vi "Compacting.vi"() -> ()   [LabVIEW 2019]
uses:
  JSONtext.lvlib
  c5c4e588-2033-429a-969a-39fff3336798.vi
  685e62f0-2af9-4f10-a6a8-997b7a51fd57.vi
  4d49a5eb-9da4-4064-b713-16a5944244b5.vi
panel:
  out "length":i32
  out "x = y?":bool
  out "Compacted":string
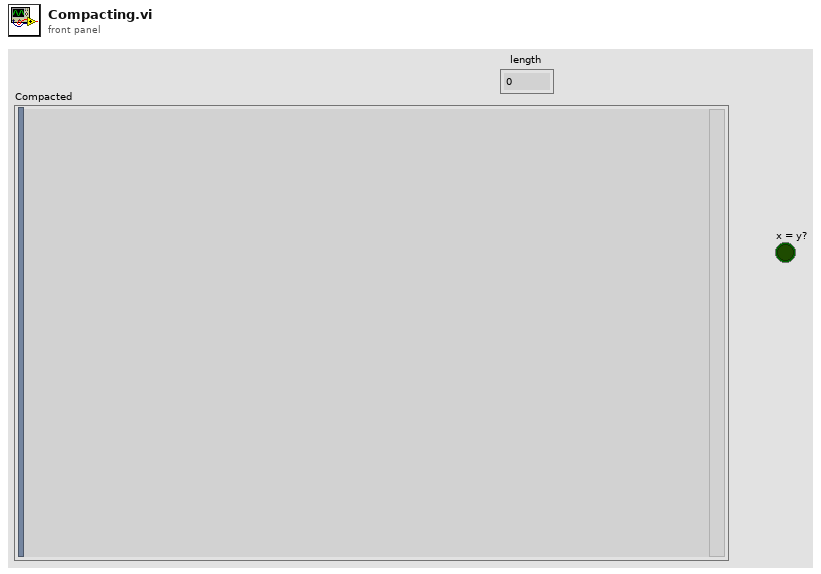
[diagram p1: front panel]
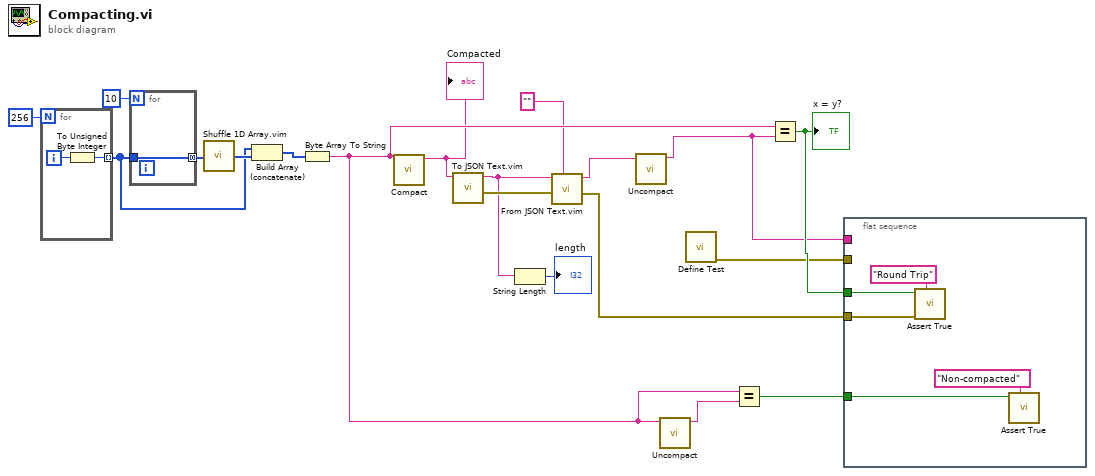
[diagram p0: block diagram]
diagram:
  n1 = for {
    N: 256 -> [_]
    tunnel: [w20] -> w4 mode=indexing
    i -> [w21]
    n2 = To Unsigned Byte Integer(number=w21) -> (unsigned 8bit integer=w20:u8)
  }
  n3 = for {
    N: 10 -> [_]
    tunnel: w4 -> [w22]
    tunnel: [w22] -> w5 mode=concatenating
  }
  n4 = call "Shuffle 1D Array.vim"("array"=w5) -> ("shuffled array"=w8:u8[])  [unwired: 4 in]
  n5 = Build Array (concatenate)(w4, w8) -> (w6:u8[])
  n6 = Byte Array To String(unsigned byte array=w6) -> (string=w16:string)
  n7 = call "Compact.vi"("Flattened Data"=w16) -> ("Compacted"=w13:string)  [unwired: 10 in]
  "Compacted" <- w13
  n8 = call "To JSON Text.vim"("Anything"=w13) -> ("error out"=w11:errorcluster, "<JSON>"=w1:string)  [unwired: 9 in]
  n9 = String Length(string=w1) -> (length=→"length":i32)
  n10 = call "From JSON Text.vim"("Data Type and Default Value"="", "error in (no error)"=w11, "JSON"=w1) -> ("error out"=w9:errorcluster, "Data out"=w12:string)  [unwired: 7 in]
  n11 = call "Uncompact.vi"("Compacted"=w12) -> ("Uncompacted"=w3:string)  [unwired: 10 in]
  n12 = call "Uncompact.vi"("Compacted"=w16) -> ("Uncompacted"=w17:string)  [unwired: 10 in]
  n13 = call <vilib>:"Define Test.vi"() -> ("error out"=w10:errorcluster)  [unwired: 11 in]
  n14 = Equal?(x=w16, y=w17) -> (x = y?=w15:bool)
  n15 = Equal?(x=w16, y=w3) -> (x = y?=w18:bool)
  "x = y?" <- w18
  n16 = flat-sequence {
    tunnel: w18 -> [w26]
    tunnel: w15 -> [w24]
    tunnel: w10 -> [_]
    tunnel: w9 -> [w23]
    tunnel: w3 -> [_]
    frame #0 {
      n17 = call <vilib>:"Assert True.vi"("Label"="Round Trip", "error in (no error)"=w23, "True?"=w26) -> ()  [unwired: 8 in, 1 out]
      n18 = call <vilib>:"Assert True.vi"("Label"="Non-compacted", "True?"=w24) -> ()  [unwired: 9 in, 1 out]
    }
  }
